vi "TcpIp_Connect.vi"(10 "Port":u16, 11 "IP":string) -> (3 "连接ID":refnum<k5>)   [LabVIEW 2013]
panel:
  out "错误输出":errorcluster
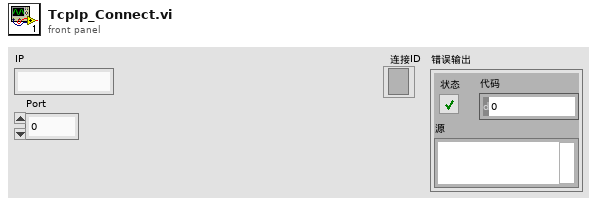
[diagram p1: front panel]
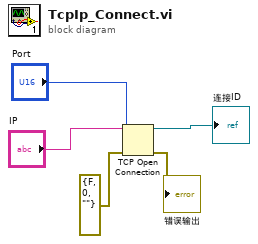
[diagram p0: block diagram]
diagram:
  n1 = TCP Open Connection(address="IP", remote port or service name="Port", error in (no error)=errorcluster {"status"=FALSE, "code"=0, "source"=""} ("错误输入（无错误）")) -> (connection ID=→"连接ID":refnum<k5>, error out=→"错误输出":errorcluster)  [unwired: 2 in]
